vi "Teststand Edit Template.vi"(8 "error in":errorcluster, 11 "Sequence Context In":refnum<k7>) -> (0 "error out":errorcluster)   [LabVIEW 2023, in "LTT_TeststandSteptypes.lvlib"]
uses:
  LTT_TeststandSteptypes.lvlib
  <vilib>/addons/TestStand/_TSUtility.llb/TestStand - Start Modal Dialog (Sequence Context).vi
  <vilib>/addons/TestStand/_TSUtility.llb/TestStand - End Modal Dialog (Sequence Context).vi
  HardwareAbstractionLayer_LVOOP/Database/Database.lvclass
  HardwareAbstractionLayer_LVOOP/Database/SQL Public VI/Control/DB Options.ctl
panel:
  in  "Close":bool
  in  "OK":bool
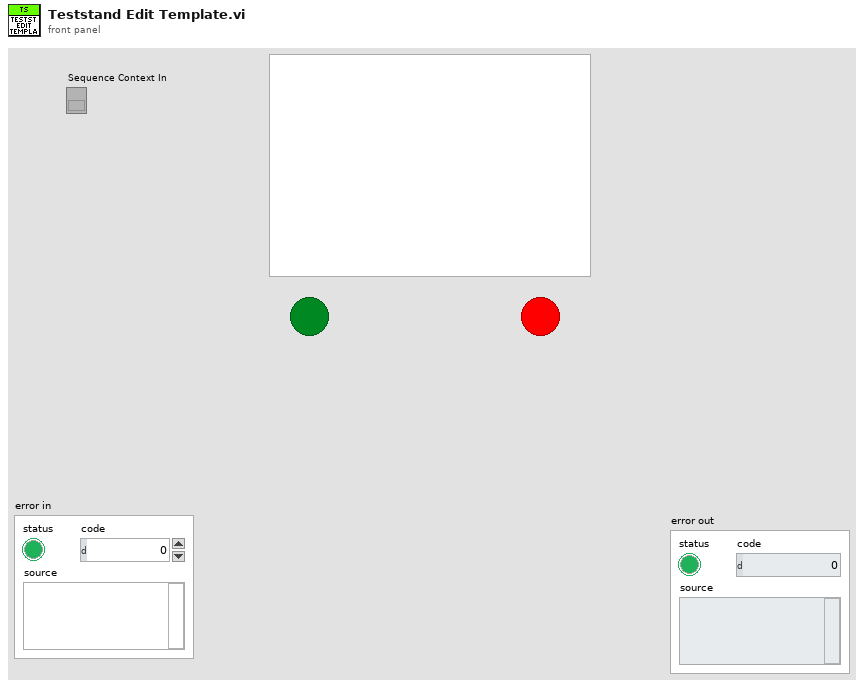
[diagram p1: front panel]
types:
  T1 = typedef "HardwareAbstractionLayer_LVOOP.lvlib/Database.lvclass/DB Options.ctl" = enum16{"Init", "Select Data", "Insert Data", "Update Data", "Delete Data", "Execute Query", "Create Schema", "Create Table", "List Tables", "List Columns", "Close"}
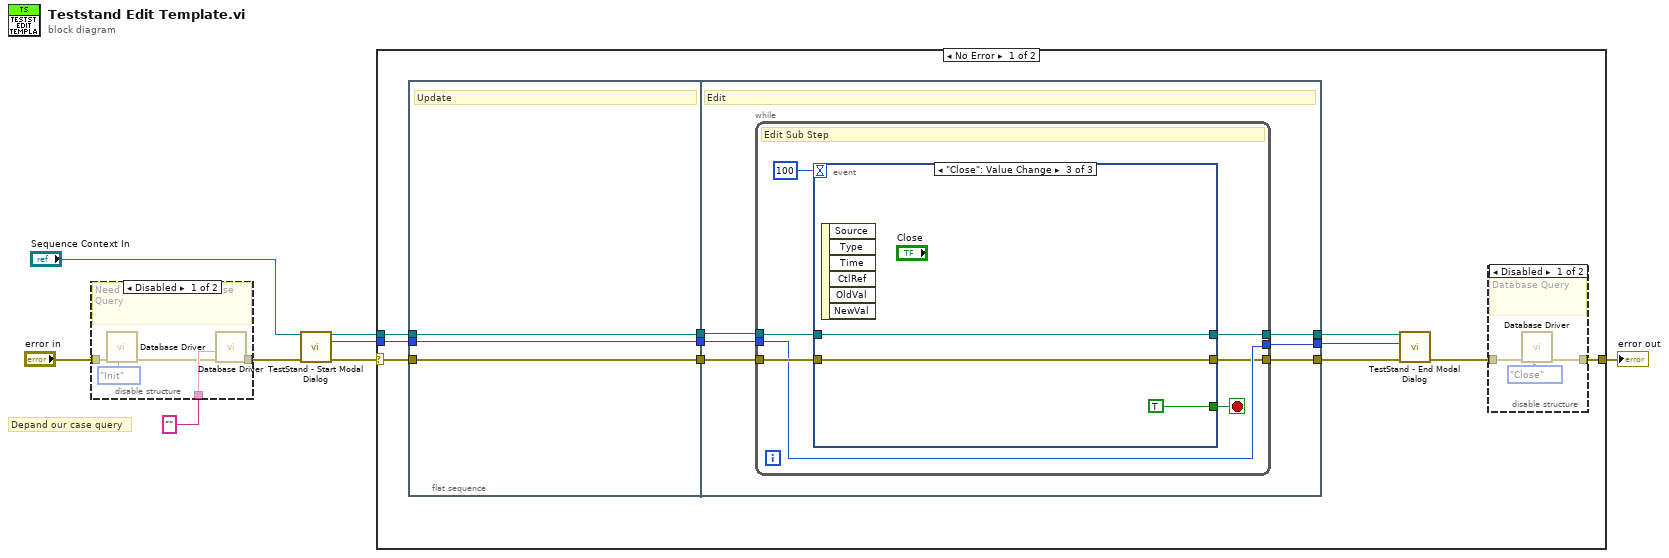
[diagram p0: block diagram]
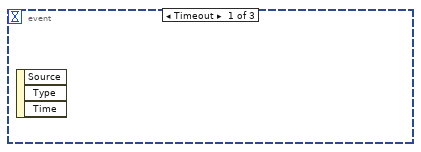
[diagram p3: hidden frame]
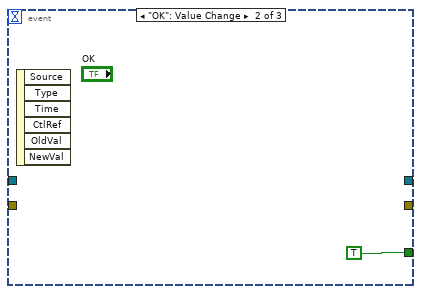
[diagram p4: hidden frame]
diagram:
  # "Depand our case query"
  n1 = disable-structure shown="Disabled" {
    disable-tunnel: "error in" -> [w13 _]
    disable-tunnel: [w12 _] -> w3
    disable-tunnel: "" ("SQL query") -> [w11 _]
    frame Disabled {
      # "Need to Enable for Database Query"
      n2 = call "Database Driver.vi"("Options"=DB_Options."Init", "error in"=w13) -> ("error out"=w10:errorcluster)  [unwired: 6 in, 3 out]
      n3 = call "Database Driver.vi"("error in"=w10, "SQL query"=w11) -> ("error out"=w12:errorcluster)  [unwired: 6 in, 3 out]
    }
    frame Enabled {
    }
  }
  n4 = call-poly <vilib>:"TestStand - Start Modal Dialog.vi"("Sequence Context In"="Sequence Context In", "error in (no error)"=w3) -> ("Sequence Context Out"=w5:refnum<k7>, "Modal ID"=w4:i32, "error out"=w6:errorcluster)  [unwired: 9 in, 2 out]
  n5 = case shown="No Error" w6 {
    selector: w6 -> [w21 w48]
    tunnel: w5 -> [w18 _]
    tunnel: w4 -> [w17 _]
    tunnel: [w14 w48] -> w1
    frame No Error {
      n6 = flat-sequence {
        tunnel: w21 -> [w30]
        tunnel: [w30] -> w24
        tunnel: w18 -> [w29]
        tunnel: w17 -> [w28]
        tunnel: [w29] -> w23
        tunnel: [w28] -> w22
        tunnel: w24 -> [w34]
        tunnel: [w32] -> w20
        tunnel: w23 -> [w36]
        tunnel: w22 -> [w35]
        tunnel: [w33] -> w16
        tunnel: [w31] -> w15
        frame #0 {
          # "Update"
        }
        frame #1 {
          # "Edit"
          n7 = while {
            tunnel: w36 -> [w41]
            tunnel: w35 -> [w38]
            tunnel: w34 -> [w39]
            tunnel: [w40] -> w31
            tunnel: [w38] -> w33
            tunnel: [w37] -> w32
            stop <- w42 stop-if-true
            # "Edit Sub Step"
            n8 = event shown="[2] \"Close\": Value Change" {
              selector: _ -> [_ _ _]
              dyn-events: _ -> [_ _ _]
              timeout: 100 -> [_ _ _]
              tunnel: [_ TRUE TRUE] -> w42
              tunnel: [_ _ w46] -> w40
              tunnel: w41 -> [_ _ w46]
              tunnel: w39 -> [_ _ w45]
              tunnel: [_ _ w45] -> w37
              event Timeout {
                n9 = event-data() -> ()  [unwired: 1 in, 3 out]
              }
              event "OK": Value Change {
                n10 = event-data() -> ()  [unwired: 1 in, 6 out]
              }
              event "Close": Value Change {
                n11 = event-data() -> ()  [unwired: 1 in, 6 out]
              }
            }
          }
        }
      }
      n12 = call-poly <vilib>:"TestStand - End Modal Dialog.vi"("Sequence Context In"=w15, "Modal ID"=w16, "error in (no error)"=w20) -> ("error out"=w19:errorcluster)  [unwired: 12 in]
      n13 = disable-structure shown="Disabled" {
        disable-tunnel: w19 -> [w27 _]
        disable-tunnel: [w26 _] -> w14
        frame Disabled {
          # "Need to Enable for Database Query"
          n14 = call "Database Driver.vi"("Options"=DB_Options."Close", "error in"=w27) -> ("error out"=w26:errorcluster)  [unwired: 6 in, 3 out]
        }
        frame Enabled {
        }
      }
    }
    frame Error {
    }
  }
  "error out" <- w1
